vi "CreateCS250-CameraHardwareObject.vi"(8 "error in (no error)":errorcluster, 11 "Photometrics_CH-250_Cam in":refnum<class "Photometrics_CH-250_Cam.lvclass">) -> (0 "error out":errorcluster, 3 "Photometrics_CH-250_Cam out":refnum<class "Photometrics_CH-250_Cam.lvclass">)   [LabVIEW 2013, in "Photometrics_CH-250_Cam.lvclass"]
uses:
  Photometrics_CH-250_Cam.lvclass
  CameraSessionClass/CS250-CameraHardwareClass.lvclass
  Photometrics_CH-250_Cam.lvclass/Photometrics_CH-250_Cam.ctl
  shared/Cameras/GenericCameraClass/GenericCamera.lvclass
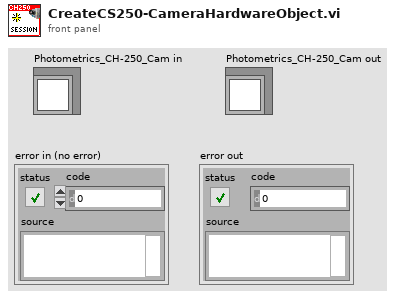
[diagram p1: front panel]
types:
  T1 = cluster{"s1":u16, "s2":u16, "sbin":u16, "p1":u16, "p2":u16, "pbin":u16}
  T2 = typedef "IMAQ Image.ctl" = refnum<image>
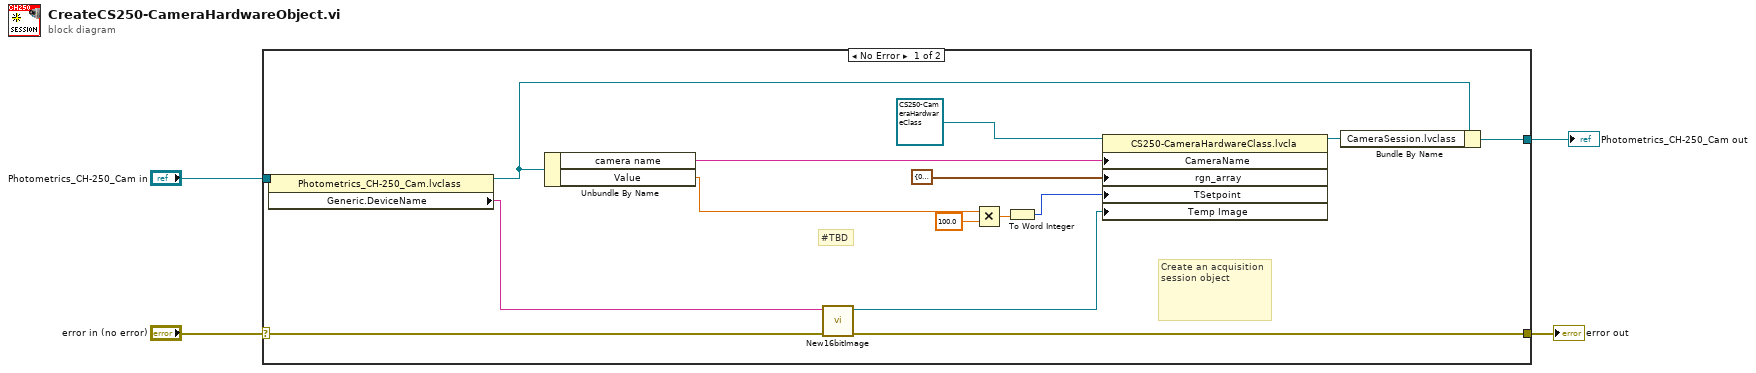
[diagram p0: block diagram]
diagram:
  n1 = case shown="No Error" "error in (no error)" {
    selector: "error in (no error)" -> [w12 w21]
    tunnel: [w19 w20] -> w4
    tunnel: "Photometrics_CH-250_Cam in" -> [w9 w20]
    tunnel: [w11 w21] -> w1
    frame No Error {
      # "#TBD"
      # "Create an acquisition session object"
      n2 = property class="Photometrics_CH-250_Cam.lvclass"(reference=w9) -> (reference out=w8:refnum<class "Photometrics_CH-250_Cam.lvclass">, "Generic.DeviceName"=w7:string)  [unwired: 1 in, 1 out]
      n3 = Unbundle By Name(w8) -> ("camera name"=w14:string, "Value"=w6:dbl)
      n4 = call "New16bitImage.vi"("error in (no error)"=w12, "ImageName"=w7) -> ("error out"=w11:errorcluster, "Refnum out"=w10:T2)  [unwired: 8 in]
      n5 = Multiply(x=w6, y=100.0) -> (x*y=w17:dbl)
      n6 = To Word Integer(number=w17) -> (16bit integer=w18:i16)
      n7 = property class="CS250-CameraHardwareClass.lvcla"(reference=refnum<class "CS250-CameraHardwareClass.lvclass"> refnum ("CameraSession in"), "CameraName"=w14, "rgn_array"=T1 {"s1"=0, "s2"=512, "sbin"=1, "p1"=0, "p2"=512, "pbin"=1}, "TSetpoint"=w18, "Temp Image"=w10) -> (reference out=w15:refnum<class "CS250-CameraHardwareClass.lvclass">)  [unwired: 1 in, 1 out]
      n8 = Bundle By Name(cluster=w8, "CameraSession.lvclass"=w15) -> (w19:refnum<class "Photometrics_CH-250_Cam.lvclass">)
    }
    frame Error {
    }
  }
  "Photometrics_CH-250_Cam out" <- w4
  "error out" <- w1
